vi "Create folder if not exists.vi"(8 "error in":errorcluster, 11 "Path in":path) -> (0 "error out":errorcluster, 3 "Path In":path, 5 "folder exists?":bool)   [LabVIEW 2013, in "FileIO lib.lvlib"]
uses:
  FileIO lib.lvlib
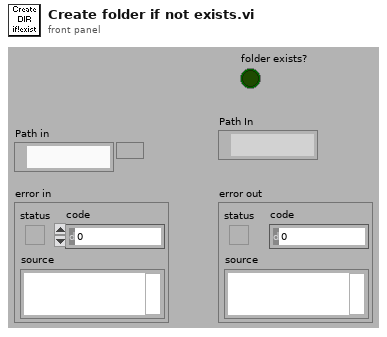
[diagram p1: front panel]
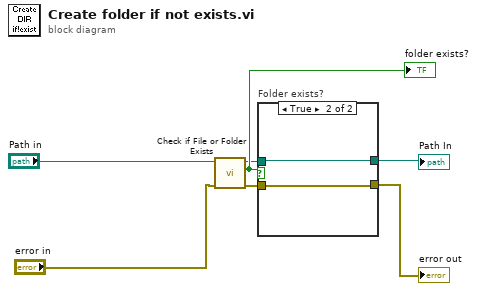
[diagram p0: block diagram]
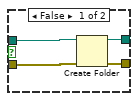
[diagram p2: hidden frame]
diagram:
  n1 = call <vilib>:"Check if File or Folder Exists.vi"("error in (no error)"="error in", "path"="Path in") -> ("error out"=w3:errorcluster, "file or folder exists?"=w7:bool, "dup path"=w4:path)  [unwired: 7 out]
  "folder exists?" <- w7
  n2 = case "Folder exists?" shown="True" w7 {
    tunnel: [w11 w13] -> w1
    tunnel: [w10 w12] -> w2
    tunnel: w3 -> [w9 w12]
    tunnel: w4 -> [w8 w13]
    frame False {
      n3 = Create Folder(path (use dialog)=w8, error in=w9) -> (created path=w11:path, error out=w10:errorcluster)  [unwired: 2 out]
    }
    frame True {
    }
  }
  "error out" <- w2
  "Path In" <- w1
